vi "Filtra misure rt.vi"(8 "open vi":bool, 10 "Riga misure RT":string[](array[string]), 11 "Col head":string[](array[string])) -> (3 "RIGA MISURA RT":string[](array[string]))   [LabVIEW 2019]
panel:
  in  "FILTRA RT":bool[](array[boolean])=[TRUE, TRUE, TRUE, TRUE, TRUE, TRUE, TRUE, TRUE, TRUE, TRUE, TRUE, TRUE, TRUE, TRUE, TRUE, TRUE, TRUE]
  # "MISURE REAL TIME"
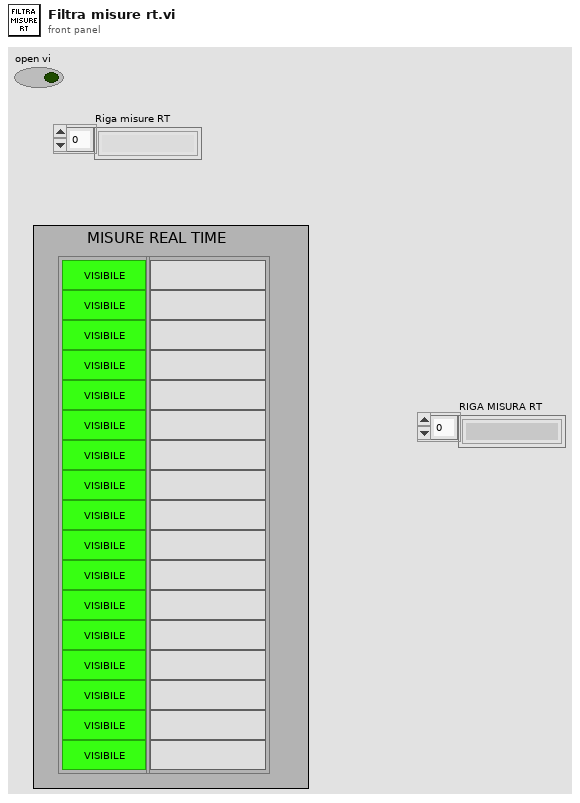
[diagram p1: front panel]
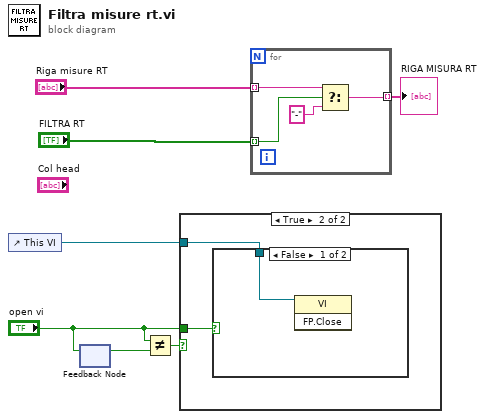
[diagram p0: block diagram]
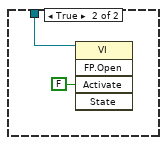
[diagram p3: hidden frame]
diagram:
  n1 = control-ref of="This VI"() -> (w4:refnum<vi>)
  n2 = feedback-in #1("open vi") -> ()
  n3 = feedback #1() -> (w3:bool)  [unwired: 1 in]
  n4 = Not Equal?(x="open vi", y=w3) -> (x != y?=w1:bool)
  n5 = case shown="True" w1 {
    tunnel: w4 -> [_ w9]
    tunnel: "open vi" -> [_ w8]
    frame False {
    }
    frame True {
      n6 = case shown="False" w8 {
        tunnel: w9 -> [w10 w12]
        frame False {
          n7 = invoke class="VI" method="FP.Close"(reference=w10) -> ()  [unwired: 2 in, 3 out]
        }
        frame True {
          n8 = invoke class="VI" method="FP.Open"(reference=w12, "Activate"=FALSE ("Activate?")) -> ()  [unwired: 3 in, 5 out]
        }
      }
    }
  }
  n9 = for {
    tunnel: "Riga misure RT" -> [w15] mode=indexing
    tunnel: "FILTRA RT" -> [w16] mode=indexing
    tunnel: [w13] -> w5 mode=indexing
    n10 = Select(t=w15, s=w16, f="-") -> (s? t:f=w13:string)
  }
  "RIGA MISURA RT" <- w5
